vi "Close Sessions AWG.vi"(8 "error in (no error)":errorcluster, 11 "Semiconductor Module Context":T1) -> (0 "error out":errorcluster)   [LabVIEW 2013]
uses:
  <vilib>/NI_TestStand_SemiconductorModule/NI_TestStand_Semiconductor_Module.lvlibp/PinMap/General/SemiconductorModuleContext.ctl
  <vilib>/NI_TestStand_SemiconductorModule/NI_TestStand_Semiconductor_Module.lvlibp
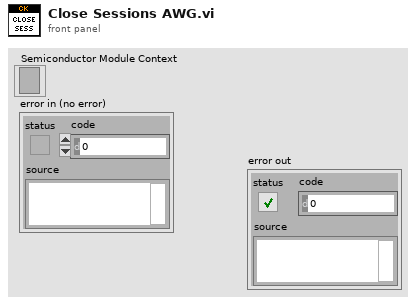
[diagram p1: front panel]
types:
  T1 = typedef "NI_TestStand_Semiconductor_Module.lvlibp/SemiconductorModuleContext.ctl" = refnum<k7>
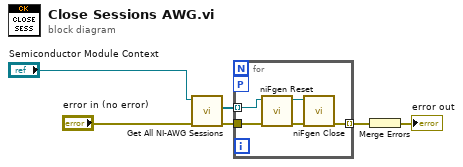
[diagram p0: block diagram]
diagram:
  n1 = call "Get All NI-AWG Sessions.vi"("error in (no error)"="error in (no error)", "Semiconductor Module Context"="Semiconductor Module Context") -> ("error out"=w3:errorcluster, "Instrument Sessions"=w4:refnum<k15>[])  [unwired: 7 in, 1 out]
  n2 = for {
    tunnel: [w11] -> w5 mode=indexing
    workers-P: _ -> [_]
    tunnel: w3 -> [w8]
    tunnel: w4 -> [w7] mode=indexing
    n3 = call <instrlib>:"niFgen Reset.vi"("error in (no error)"=w8, "Instrument Handle"=w7) -> ("error out"=w10:errorcluster, "Instrument Handle Out"=w9:refnum<k15>)  [unwired: 8 in]
    n4 = call <instrlib>:"niFgen Close.vi"("error in (no error)"=w10, "Instrument Handle"=w9) -> ("error out"=w11:errorcluster)  [unwired: 9 in]
  }
  n5 = Merge Errors(w5) -> (→"error out":errorcluster)
